vi "SeqnWrite.vi"(8 "error in (no error)":errorcluster, 10 "Seqn in":refnum<class "Sequence.lvclass">, 11 "File in":path) -> (0 "error out":errorcluster)   [LabVIEW 2012, in "Sequence.lvclass"]
uses:
  Sequence.lvclass
  Cohort.lvclass
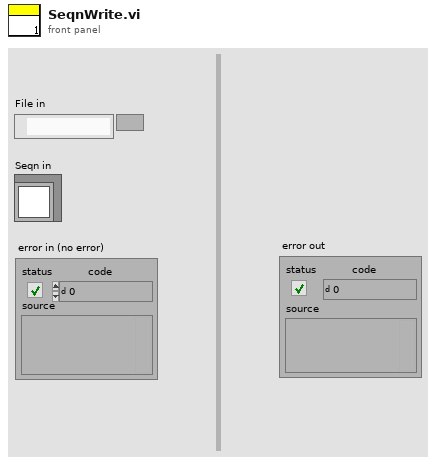
[diagram p1: front panel]
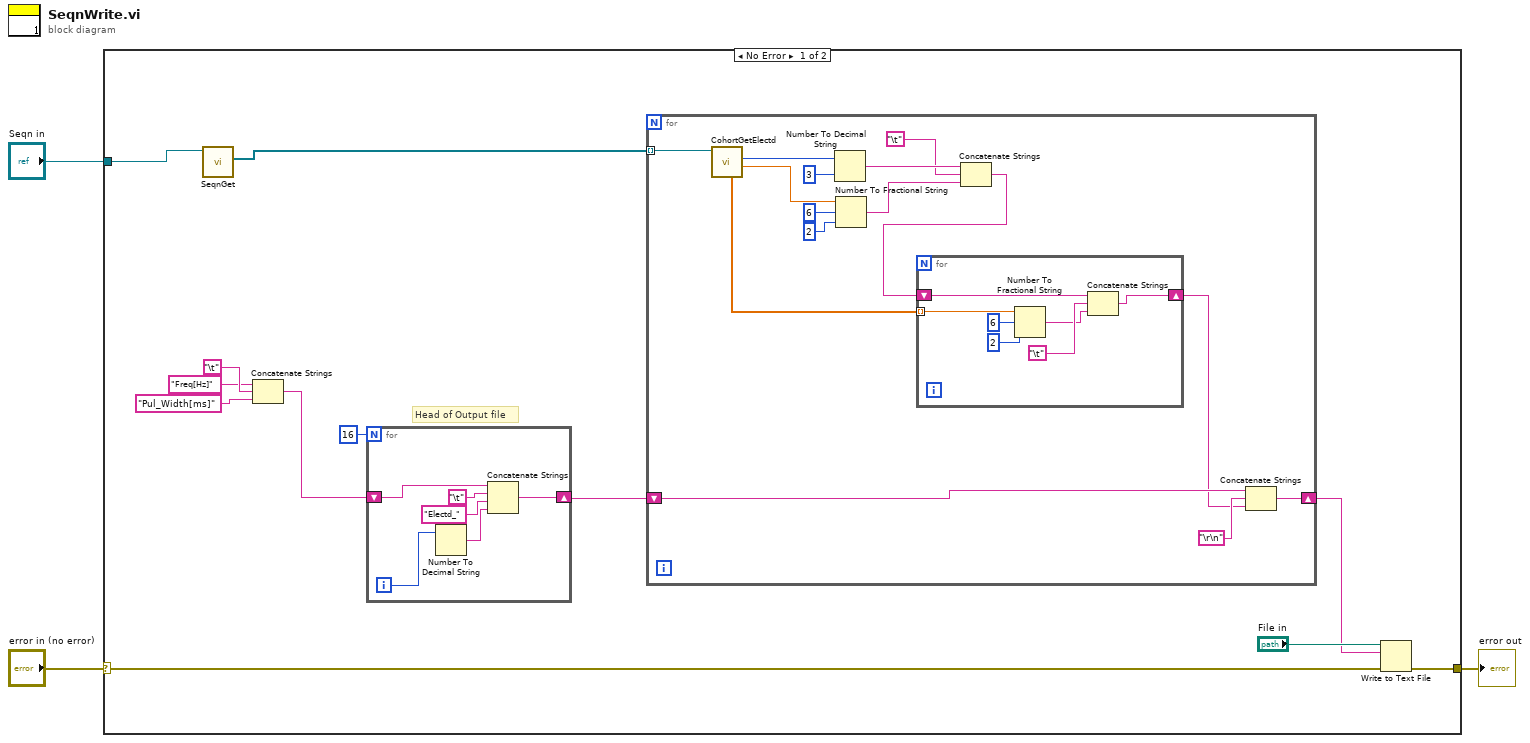
[diagram p0: block diagram]
diagram:
  n1 = case shown="No Error" "error in (no error)" {
    selector: "error in (no error)" -> [w12 w44]
    tunnel: "Seqn in" -> [w15 _]
    tunnel: [w13 w44] -> w2
    frame No Error {
      # "Head of Output file"
      n2 = call-dynamic "SeqnGet.vi"("Sequence in"=w15) -> ("Cohorts"=w14:refnum<class "Cohort.lvclass">[])  [unwired: 8 in, 2 out]
      n3 = Concatenate Strings("Freq[Hz]", "\t", "Pul_Width[ms]") -> (w5:string)
      n4 = for {
        N: 16 -> [_]
        shift-right: [w18] -> w6
        shift-left: w5 -> [w17]
        i -> [w16]
        n5 = Number To Decimal String(number=w16) -> (decimal integer string=w19:string)  [unwired: 1 in]
        n6 = Concatenate Strings(w17, "\t", "Electd_", w19) -> (w18:string)
      }
      n7 = for {
        tunnel: w14 -> [w36] mode=indexing
        shift-right: [w24] -> w10
        shift-left: w6 -> [w25]
        n8 = call-dynamic "CohortGetElectd.vi"("Cohort in"=w36) -> ("Pulse Width [s]"=w33:sgl, "Pulse Frequency [Hz]"=w35:u8, "Amplitude"=w30:sgl[])  [unwired: 7 in, 1 out]
        n9 = Number To Decimal String(number=w35, width (-)=i16 3) -> (decimal integer string=w29:string)
        n10 = Number To Fractional String(number=w33, width (-)=i16 6, precision (6)=i16 2) -> (F-format string=w28:string)  [unwired: 1 in]
        n11 = Concatenate Strings(w29, "\t", w28) -> (w26:string)
        n12 = for {
          tunnel: w30 -> [w43] mode=indexing
          shift-right: [w40] -> w22
          shift-left: w26 -> [w39]
          n13 = Number To Fractional String(number=w43, width (-)=i16 6, precision (6)=i16 2) -> (F-format string=w37:string)  [unwired: 1 in]
          n14 = Concatenate Strings(w39, "\t", w37) -> (w40:string)
        }
        n15 = Concatenate Strings(w25, "\r\n", w22) -> (w24:string)
      }
      n16 = Write to Text File(file (use dialog)="File in", text=w10, error in=w12) -> (error out=w13:errorcluster)  [unwired: 1 in, 2 out]
    }
    frame Error {
    }
  }
  "error out" <- w2
